vi "SetMaxCurrent.vi"(8 "error in (no error)":errorcluster, 11 "Laser Diode Controller in":refnum<class "KLD101.lvclass">) -> (0 "error out":errorcluster, 3 "Laser Diode Controller out":refnum<class "KLD101.lvclass">)   [LabVIEW 2016, in "Laser Diode Controller.lvlib" / "KLD101.lvclass"]
uses:
  KLD101.lvclass
  KLD101.lvclass/KLD101.ctl
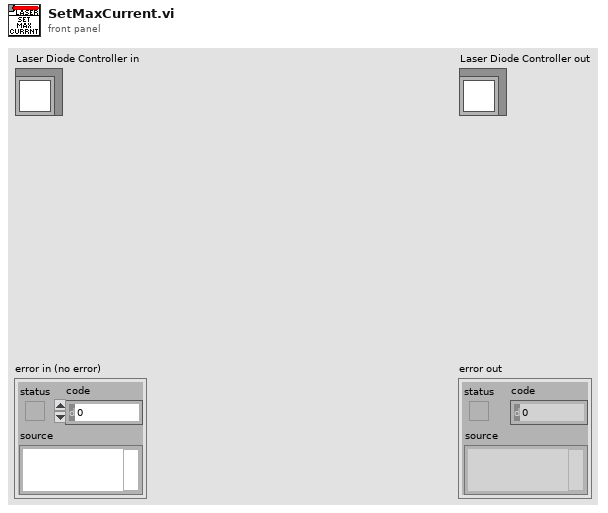
[diagram p1: front panel]
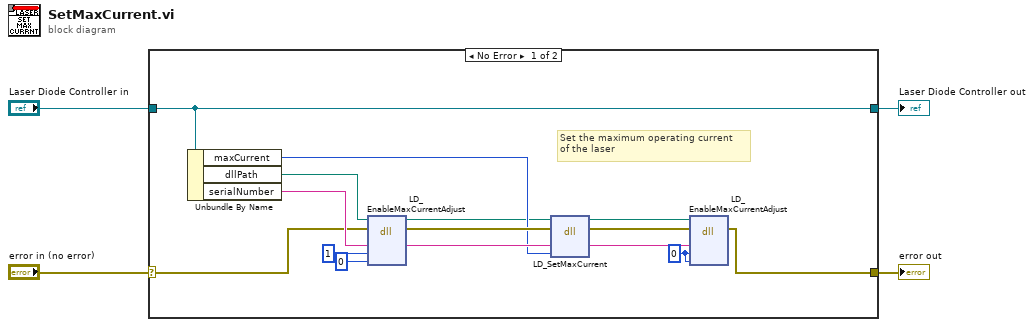
[diagram p0: block diagram]
diagram:
  n1 = case shown="No Error" "error in (no error)" {
    selector: "error in (no error)" -> [w11 w21]
    tunnel: [w17 w21] -> w3
    tunnel: [w19 w20] -> w1
    tunnel: "Laser Diode Controller in" -> [w19 w20]
    frame No Error {
      w15 = u8 0 ("enableAdjust")
      # "Set the maximum operating current\nof the laser"
      n2 = Unbundle By Name(w19) -> ("maxCurrent"=w8:i16, "dllPath"=w7:path, "serialNumber"=w12:string)
      n3 = dll-call lib="C:/IDEXX Software/Collimation/data/Thorlabs.MotionControl.KCube.LaserDiode.dll" fn="LD_EnableMaxCurrentAdjust"(path in=w7, error in=w11, "serialNumber"=w12, "enableAdjust"=u8 1, "enableDiode"=u8 0) -> (path out=w6:path, error out=w10:errorcluster, "serialNumber"=w13:string)  [unwired: 4 in]
      n4 = dll-call lib="C:/IDEXX Software/Collimation/data/Thorlabs.MotionControl.KCube.LaserDiode.dll" fn="LD_SetMaxCurrent"(path in=w6, error in=w10, "serialNumber"=w13, "maxCurrent"=w8) -> (path out=w5:path, error out=w18:errorcluster, "serialNumber"=w16:string)  [unwired: 3 in]
      n5 = dll-call lib="C:/IDEXX Software/Collimation/data/Thorlabs.MotionControl.KCube.LaserDiode.dll" fn="LD_EnableMaxCurrentAdjust"(path in=w5, error in=w18, "serialNumber"=w16, "enableAdjust"=w15, "enableDiode"=w15) -> (error out=w17:errorcluster)  [unwired: 5 in, 1 out]
    }
    frame Error {
    }
  }
  "error out" <- w3
  "Laser Diode Controller out" <- w1
